vi "Read hSession.vi"(8 "error in (no error)":errorcluster, 11 "Session HVPS in":refnum<class "Session HVPS.lvclass">) -> (0 "error out":errorcluster, 2 "Session Handle":T1, 3 "Session HVPS out":refnum<class "Session HVPS.lvclass">)   [LabVIEW 2013, in "Session HVPS.lvclass"]
uses:
  Session HVPS.lvclass
  <userlib>/_Session Fwk/Typedefs/Session Handle.ctl
  <userlib>/_Session Fwk/Session - Root.lvclass
  Session HVPS.lvclass/Session HVPS.ctl
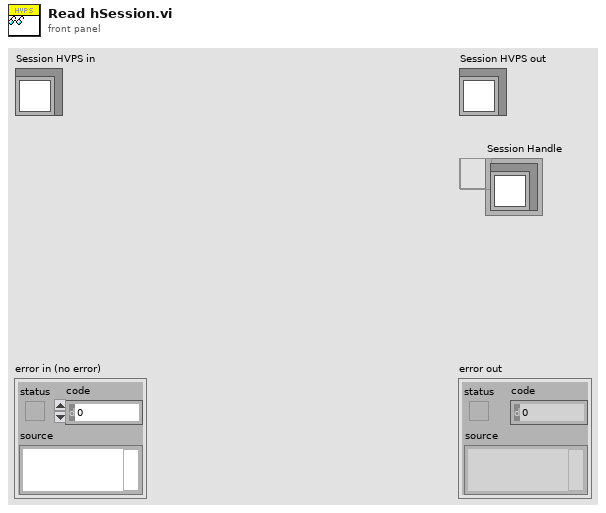
[diagram p1: front panel]
types:
  T1 = typedef "Session - Root.lvclass/Session Handle.ctl" = refnum<data-value>
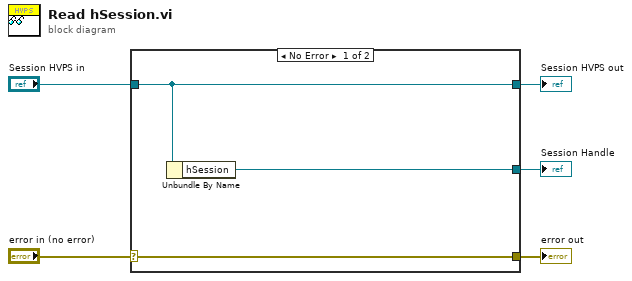
[diagram p0: block diagram]
diagram:
  n1 = case shown="No Error" "error in (no error)" {
    selector: "error in (no error)" -> [w8 w9]
    tunnel: [w8 w9] -> w4
    tunnel: [w7 w10] -> w2
    tunnel: "Session HVPS in" -> [w7 w10]
    tunnel: [w6 _] -> w1
    frame No Error {
      n2 = Unbundle By Name(w7) -> ("hSession"=w6:T1)
    }
    frame Error {
    }
  }
  "error out" <- w4
  "Session HVPS out" <- w2
  "Session Handle" <- w1
